vi "readCOM_Data.vi"() -> ()   [LabVIEW 2020]
uses:
  <vilib>/Instr/_visa.llb/VISA Configure Serial Port (Instr).vi
panel:
  out "Array":string[](array[string])
  out "Loop Time [ms]":u32
  in  "stop":bool
  out "Serial Settings:Number of Bytes at Serial Port":u32
  in  "baud rate (9600)":u32=9600
  in  "VISA resource name":refnum<visa-resource-name>
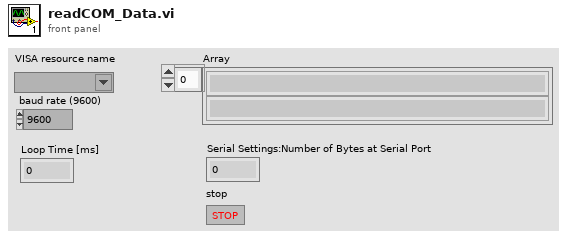
[diagram p1: front panel]
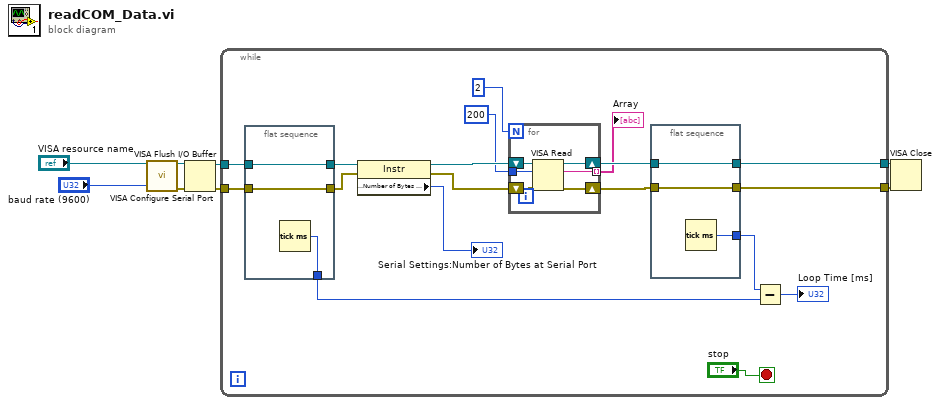
[diagram p0: block diagram]
diagram:
  n1 = call-poly "VISA Configure Serial Port"("VISA resource name"="VISA resource name", "baud rate (9600)"="baud rate (9600)") -> ("VISA resource name out"=w5:refnum<visa-resource-name>, "error out"=w6:errorcluster)  [unwired: 12 in]
  n2 = VISA Flush I/O Buffer(VISA resource name=w5, error in (no error)=w6) -> (VISA resource name out=w3:refnum<visa-resource-name>, error out=w4:errorcluster)  [unwired: 1 in]
  n3 = while {
    tunnel: w4 -> [w26]
    tunnel: w3 -> [w25]
    tunnel: [w17] -> w2
    tunnel: [w16] -> w1
    stop <- "stop" stop-if-true
    n4 = flat-sequence {
      tunnel: w26 -> [w38]
      tunnel: w25 -> [w37]
      tunnel: [w38] -> w23
      tunnel: [w37] -> w24
      tunnel: [w36] -> w13
      frame #0 {
        n5 = Tick Count (ms)() -> (millisecond timer value=w36:u32)
      }
    }
    n6 = property class="Instr"(reference=w24, error in=w23) -> (reference out=w22:refnum<visa-resource-name>, error out=w21:errorcluster, "Serial Settings:Number of Bytes at Serial Port"=→"Serial Settings:Number of Bytes at Serial Port":u32)
    n7 = for {
      N: 2 -> [_]
      tunnel: 200 -> [w28]
      shift-right: [w29] -> w15
      shift-left: w22 -> [w32]
      shift-right: [w30] -> w18
      shift-left: w21 -> [w31]
      tunnel: [w27] -> w10 mode=indexing
      n8 = VISA Read(VISA resource name=w32, byte count=w28, error in (no error)=w31) -> (VISA resource name out=w29:refnum<visa-resource-name>, read buffer=w27:string, error out=w30:errorcluster)  [unwired: 1 out]
    }
    "Array" <- w10
    n9 = flat-sequence {
      tunnel: w18 -> [w35]
      tunnel: w15 -> [w34]
      tunnel: [w35] -> w17
      tunnel: [w34] -> w16
      tunnel: [w33] -> w14
      frame #0 {
        n10 = Tick Count (ms)() -> (millisecond timer value=w33:u32)
      }
    }
    n11 = Subtract(x=w14, y=w13) -> (x-y=→"Loop Time [ms]":u32)
  }
  n12 = VISA Close(VISA resource name=w1, error in (no error)=w2) -> ()  [unwired: 1 out]
